vi "Read Attribute.vi"(9 "Type":variant, 10 "Name":string, 11 "Executioner in":refnum<class "Executioner.lvclass">) -> (1 "Value":variant, 2 "Found?":bool, 3 "Executioner out":refnum<class "Executioner.lvclass">)   [LabVIEW 2020, in "Test Executive.lvlib" / "Executioner.lvclass"]
uses:
  <vilib>/gpm_packages/@cs/test-executive/Source/Test Executive/Executioner/Executioner.lvclass
  <vilib>/gpm_packages/@cs/test-executive/Source/Test Executive/Executioner/Executioner.lvclass/Executioner.ctl
  <vilib>/gpm_packages/@cs/lookup-table/Source/LookupTable/LookupTable.lvclass/LookupTable.ctl
  efd395ac-eb41-409b-8349-64ddd86dcdd7.vi
  <vilib>/gpm_packages/@cs/lookup-table/Source/LookupTable/Read Table Reference.vi
  efd395ac-eb41-409b-8349-64ddd86dcdd7.vi/b78a388c-1bb7-44ee-b536-08e529786940.vi
  <vilib>/gpm_packages/@cs/lookup-table/Source/LookupTable/LookupTable.lvclass
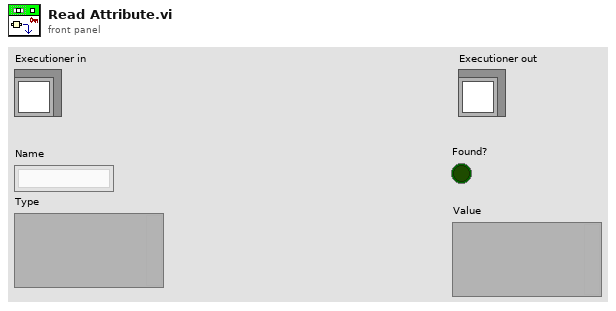
[diagram p1: front panel]
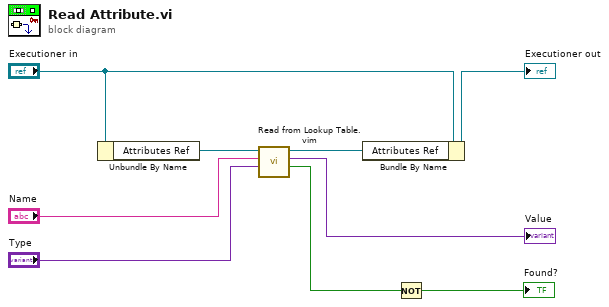
[diagram p0: block diagram]
diagram:
  n1 = Unbundle By Name("Executioner in") -> ("Attributes Ref"=w1:refnum<data-value>)
  n2 = call "Read from Lookup Table.vim"("Type"="Type", "Item Name"="Name", "LookupTable Reference"=w1) -> ("Not Found?"=w7:bool, "Value"=→"Value":variant, "LookupTable Reference Out"=w3:refnum<data-value>)  [unwired: 5 in, 1 out]
  n3 = Bundle By Name(cluster="Executioner in", "Attributes Ref"=w3) -> (→"Executioner out":refnum<class "Executioner.lvclass">)
  n4 = Not(x=w7) -> (.not. x?=→"Found?":bool)
